vi "IndexArray.vi"() -> ()   [LabVIEW 2019]
panel:
  out "Row 0":dbl[](array[numeric])
  out "Column 0":dbl[](array[numeric])
  out "element (2x1)":dbl
  out "element (1x1)":dbl
  in  "b":dbl[][](array[numeric])
  out "element 4th Index":dbl
  out "element 1st Index":dbl
  in  "a":dbl[](array[numeric])
  # "0"
  # "1"
  # "2"
  # "Columns"
  # "0"
  # "Rows"
  # "1"
  # "2"
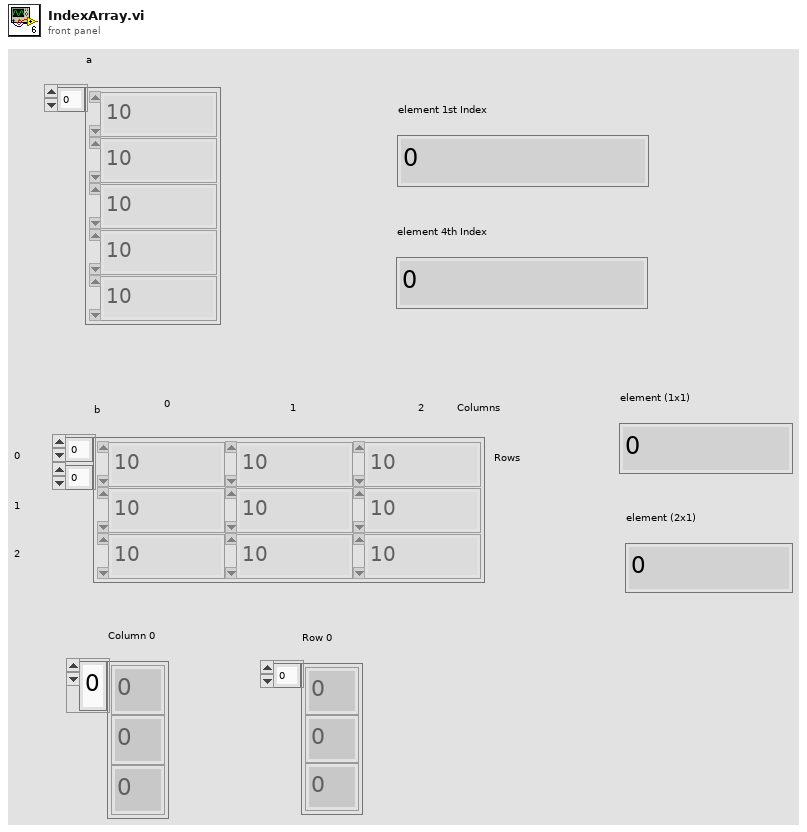
[diagram p1: front panel]
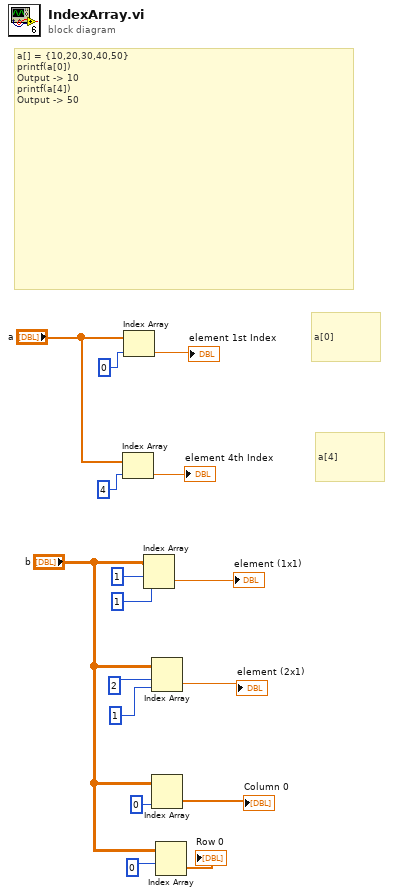
[diagram p0: block diagram]
diagram:
  # "a[4]"
  # "a[0]"
  # "a[] = {10,20,30,40,50}\nprintf(a[0])\nOutput -> 10\nprintf(a[4])\nOutput -> 50"
  n1 = Index Array(array="a", index=4) -> (element=→"element 4th Index":dbl)
  n2 = Index Array(array="a", index=0) -> (element=→"element 1st Index":dbl)
  n3 = Index Array(array="b", index (row)=1, index (col)=1 ("disabled index (col)")) -> (element=→"element (1x1)":dbl)
  n4 = Index Array(array="b", index (row)=2, index (col)=1 ("disabled index (col)")) -> (element=→"element (2x1)":dbl)
  n5 = Index Array(array="b", index (col)=0 ("disabled index (col)")) -> (element=→"Column 0":dbl[])  [unwired: 1 in]
  n6 = Index Array(array="b", index (row)=0 ("disabled index (col)")) -> (element=→"Row 0":dbl[])  [unwired: 1 in]
